vi "SE5082_Scaler.vi"(4 "Channel":u16(ring) items=["Channel 1", "Channel 2"], 8 "error in":errorcluster, 9 "Voffset":dbl, 10 "Vpp":dbl=1.0, 11 "VISA resource name in":refnum<visa-resource-name>="USB0::0x168C::0x5082::0000217419::INSTR") -> (0 "error out":errorcluster, 3 "VISA resource name out":refnum<visa-resource-name>="USB0::0x168C::0x5082::0000217419::INSTR")   [LabVIEW 2017]
uses:
  Software/Rydberg_Control/TypeDefinition/variables.ctl
panel:
  in  "HV_HI":string="200"
  in  "HV_LO":string="-100"
  in  "Readout status?":bool
  in  "Read-out commands":string[](array[string])=[":INST 1;:VOLT?", ":INST 1;:VOLT:OFFS?", ":INST 1;:OUTP?", ":INST 2;:VOLT?", ":INST 2;:VOLT:OFFS?", ":INST 2;:OUTP?"]
  out "Input waveform commands":string[](array[string])=[":INST 1;:OUTP OFF", ":INST 2;:OUTP OFF", ":INST 1;:VOLT  1.000000", ":INST 1;:VOLT:OFFS  -1.000000 "]
  out "Status output":string[](array[string])=["1.000e+00\n", "0.000e+00\n", "OFF\n", "5.000e-01\n", "0.000e+00\n", "OFF\n"]
  in  "Debug commands":string=":SOUR1:VOLT:OFFS 1\n:SOUR1:VOLT 6"
  in  "Variables":T1=[{"Value"=10.0, "Variable"="dummy", "Save with Image"=FALSE}, {"Value"=-0.0001, "Variable"="HI", "Save with Image"=FALSE}, {"Value"=-0.0002, "Variable"="LO", "Save with Image"=FALSE}, {"Value"=0.0, "Variable"="dummy1", "Save with Image"=FALSE}, {"Value"=0.0, "Variable"="dummy2", "Save with Image"=FALSE}, {"Value"=0.0, "Variable"="dummy3", "Save with Image"=FALSE}, {"Value"=0.0, "Variable"="tLEDuv", "Save with Image"=FALSE}, {"Value"=1000.0, "Variable"="tMOT0", "Save with Image"=FALSE}, {"Value"=20.0, "Variable"="tMOT1", "Save with Image"=FALSE}, {"Value"=40.0, "Variable"="tMOT2", "Save with Image"=FALSE}, {"Value"=50.0, "Variable"="tMOT3", "Save with Image"=FALSE}, {"Value"=13.0, "Variable"="tMOT3delayREP", "Save with Image"=FALSE}, {"Value"=0.05, "Variable"="tREP", "Save with Image"=FALSE}, {"Value"=0.75, "Variable"="dMOT0", "Save with Image"=FALSE}, {"Value"=1.75, "Variable"="dMOT1", "Save with Image"=FALSE}, {"Value"=1.75, "Variable"="dMOT2", "Save with Image"=FALSE}, {"Value"=0.0, "Variable"="dummy5", "Save with Image"=FALSE}, {"Value"=1.45, "Variable"="pMOT0", "Save with Image"=FALSE}, {"Value"=1.45, "Variable"="pMOT1", "Save with Image"=FALSE}, {"Value"=1.25, "Variable"="pMOT2", "Save with Image"=FALSE}, {"Value"=-1.0, "Variable"="dummy6", "Save with Image"=FALSE}, {"Value"=1.6, "Variable"="pRP0", "Save with Image"=FALSE}, {"Value"=1.6, "Variable"="pRP1", "Save with Image"=FALSE}, {"Value"=0.8, "Variable"="pRP2", "Save with Image"=FALSE}, {"Value"=0.0, "Variable"="MOTdummy0", "Save with Image"=FALSE}, {"Value"=-1.0, "Variable"="MOTdummy1", "Save with Image"=FALSE}, {"Value"=0.0, "Variable"="MOTdummy2", "Save with Image"=FALSE}, {"Value"=0.0, "Variable"="MOTdummy3", "Save with Image"=FALSE}, {"Value"=0.0, "Variable"="MOTdummy4", "Save with Image"=FALSE}, {"Value"=1.8, "Variable"="pCROSS0", "Save with Image"=FALSE}, {"Value"=1.29, "Variable"="pCROSS1", "Save with Image"=FALSE}, {"Value"=1.05, "Variable"="pCROSS2", "Save with Image"=FALSE}, {"Value"=0.75, "Variable"="pCROSS3", "Save with Image"=FALSE}, {"Value"=0.0, "Variable"="pCROSS4", "Save with Image"=FALSE}, {"Value"=5.0, "Variable"="pDIMPL0", "Save with Image"=FALSE}, {"Value"=4.4, "Variable"="pDIMPL1", "Save with Image"=FALSE}, {"Value"=3.65, "Variable"="pDIMPL2", "Save with Image"=FALSE}, {"Value"=3.55, "Variable"="pDIMPL3", "Save with Image"=FALSE}, {"Value"=3.45, "Variable"="pDIMPL4", "Save with Image"=FALSE}, {"Value"=1.8, "Variable"="pTightTrap", "Save with Image"=FALSE}, {"Value"=400.0, "Variable"="tHOLD", "Save with Image"=FALSE}, {"Value"=740.0, "Variable"="tEVAP1", "Save with Image"=FALSE}, {"Value"=2900.0, "Variable"="tEVAP2", "Save with Image"=FALSE}, {"Value"=590.0, "Variable"="tEVAP3", "Save with Image"=FALSE}, {"Value"=50.0, "Variable"="tEVAP4", "Save with Image"=FALSE}, {"Value"=50.0, "Variable"="tHOLDTight", "Save with Image"=FALSE}, {"Value"=0.0, "Variable"="ODTdummy1", "Save with Image"=FALSE}, {"Value"=0.0, "Variable"="ODTdummy2", "Save with Image"=FALSE}, {"Value"=0.0, "Variable"="ODTdummy3", "Save with Image"=FALSE}, {"Value"=0.0, "Variable"="ODTdummy4", "Save with Image"=FALSE}, {"Value"=0.0, "Variable"="ODTdummy5", "Save with Image"=FALSE}, {"Value"=3.59, "Variable"="dIMGx", "Save with Image"=FALSE}, {"Value"=3.59, "Variable"="dIMGx0", "Save with Image"=FALSE}, {"Value"=1.38, "Variable"="dIMGz", "Save with Image"=FALSE}, {"Value"=1.98, "Variable"="dEXCz", "Save with Image"=FALSE}, {"Value"=3.0, "Variable"="pABSx", "Save with Image"=FALSE}, {"Value"=1.35, "Variable"="pABSz", "Save with Image"=FALSE}, {"Value"=0.55, "Variable"="pEXCz", "Save with Image"=FALSE}, {"Value"=0.0, "Variable"="TOF", "Save with Image"=FALSE}, {"Value"=10.0, "Variable"="TOFatomFall", "Save with Image"=FALSE}, {"Value"=0.012, "Variable"="tEXP", "Save with Image"=FALSE}, {"Value"=0.2, "Variable"="tEXP2", "Save with Image"=FALSE}, {"Value"=0.082, "Variable"="tEXC", "Save with Image"=FALSE}, {"Value"=0.001, "Variable"="tWaitIoniz", "Save with Image"=FALSE}, {"Value"=0.065, "Variable"="tCAM", "Save with Image"=FALSE}, {"Value"=200.0, "Variable"="tCAMguppy", "Save with Image"=FALSE}, {"Value"=50.0, "Variable"="tCAMreadout", "Save with Image"=FALSE}, {"Value"=-0.002, "Variable"="tTrigDelay", "Save with Image"=FALSE}, {"Value"=0.0, "Variable"="tTrans", "Save with Image"=FALSE}, {"Value"=1.0, "Variable"="tEXCres", "Save with Image"=FALSE}, {"Value"=0.004, "Variable"="tPUMP", "Save with Image"=FALSE}, {"Value"=2.0, "Variable"="pBLUEswitch", "Save with Image"=FALSE}, {"Value"=2.0, "Variable"="pBLUEswitchEIT", "Save with Image"=FALSE}, {"Value"=3.5, "Variable"="dBLUE", "Save with Image"=FALSE}, {"Value"=3.5, "Variable"="dBLUE0", "Save with Image"=FALSE}, {"Value"=1.7, "Variable"="dBLUEdec", "Save with Image"=FALSE}, {"Value"=2.5, "Variable"="dBLUEdec0", "Save with Image"=FALSE}, {"Value"=3.2, "Variable"="dIMPnew", "Save with Image"=FALSE}, {"Value"=1.0, "Variable"="blueON1", "Save with Image"=FALSE}, {"Value"=0.0, "Variable"="blueON2", "Save with Image"=FALSE}, {"Value"=1.0, "Variable"="blueEXCON1", "Save with Image"=FALSE}, {"Value"=0.0, "Variable"="blueEXCON2", "Save with Image"=FALSE}, {"Value"=35.637858, "Variable"="dRydMW", "Save with Image"=FALSE}, {"Value"=16.0, "Variable"="pRydMW", "Save with Image"=FALSE}, {"Value"=50.0, "Variable"="MWduration", "Save with Image"=FALSE}, {"Value"=4.33, "Variable"="bmw0", "Save with Image"=FALSE}, {"Value"=0.02, "Variable"="bmw1", "Save with Image"=FALSE}, {"Value"=0.0, "Variable"="MWdummy1", "Save with Image"=FALSE}, {"Value"=0.0, "Variable"="MWdummy2", "Save with Image"=FALSE}, {"Value"=0.0, "Variable"="MWdummy3", "Save with Image"=FALSE}, {"Value"=4.3, "Variable"="foffset", "Save with Image"=FALSE}, {"Value"=8.64, "Variable"="fdx", "Save with Image"=FALSE}, {"Value"=-5.78, "Variable"="fdy", "Save with Image"=FALSE}, {"Value"=4.0, "Variable"="fdz", "Save with Image"=FALSE}, {"Value"=300.0, "Variable"="CH203", "Save with Image"=FALSE}, {"Value"=160.0, "Variable"="CH215", "Save with Image"=FALSE}, {"Value"=4.0, "Variable"="CH302", "Save with Image"=FALSE}, {"Value"=280.0, "Variable"="CH315", "Save with Image"=FALSE}, {"Value"=0.0, "Variable"="CH202", "Save with Image"=FALSE}, {"Value"=0.0, "Variable"="CH308", "Save with Image"=FALSE}, {"Value"=0.0, "Variable"="EFIELDdummy2", "Save with Image"=FALSE}, {"Value"=0.0, "Variable"="EFIELDdummy3", "Save with Image"=FALSE}, {"Value"=0.0, "Variable"="EFIELDdummy4", "Save with Image"=FALSE}, {"Value"=0.0, "Variable"="EFIELDdummy5", "Save with Image"=FALSE}, {"Value"=0.0, "Variable"="EFIELDdummy6", "Save with Image"=FALSE}, {"Value"=0.0, "Variable"="EFIELDdummy7", "Save with Image"=FALSE}, {"Value"=1.25, "Variable"="bMOT0", "Save with Image"=FALSE}, {"Value"=2.5, "Variable"="bMOT1", "Save with Image"=FALSE}, {"Value"=2.5, "Variable"="bMOT2", "Save with Image"=FALSE}, {"Value"=1.25, "Variable"="bMOT3", "Save with Image"=FALSE}, {"Value"=0.0, "Variable"="bCOMPx", "Save with Image"=FALSE}, {"Value"=1.35, "Variable"="bCOMPy", "Save with Image"=FALSE}, {"Value"=0.27, "Variable"="bCOMPz", "Save with Image"=FALSE}, {"Value"=0.7, "Variable"="bCOMPx1", "Save with Image"=FALSE}, {"Value"=1.1, "Variable"="bCOMPy1", "Save with Image"=FALSE}, {"Value"=0.5, "Variable"="bCOMPz1", "Save with Image"=FALSE}, {"Value"=4.35, "Variable"="bxfinal", "Save with Image"=FALSE}, {"Value"=0.0, "Variable"="byfinal", "Save with Image"=FALSE}, {"Value"=0.0, "Variable"="bzfinal", "Save with Image"=FALSE}, {"Value"=0.0, "Variable"="BFIELDdummy1", "Save with Image"=FALSE}, {"Value"=0.0, "Variable"="BFIELDdummy2", "Save with Image"=FALSE}, {"Value"=0.0, "Variable"="BFIELDdummy3", "Save with Image"=FALSE}, {"Value"=10.0, "Variable"="tCOILsettle", "Save with Image"=FALSE}, {"Value"=0.0, "Variable"="tRemove", "Save with Image"=FALSE}, {"Value"=3.6, "Variable"="pRemove", "Save with Image"=FALSE}, {"Value"=3.1, "Variable"="dF2CLEAN1x", "Save with Image"=FALSE}, {"Value"=20.0, "Variable"="tF2CLEAN1x", "Save with Image"=FALSE}, {"Value"=4.0, "Variable"="tF2CLEAN2x", "Save with Image"=FALSE}, {"Value"=0.0, "Variable"="tDelayDown", "Save with Image"=FALSE}, {"Value"=156.0, "Variable"="oDDSbluePro", "Save with Image"=FALSE}, {"Value"=-10.25, "Variable"="dDDSbluePro", "Save with Image"=FALSE}, {"Value"=50.0, "Variable"="tRampDDSbluePro", "Save with Image"=FALSE}, {"Value"=416.6261, "Variable"="oDDSred", "Save with Image"=FALSE}, {"Value"=-50.25, "Variable"="dDDSred", "Save with Image"=FALSE}, {"Value"=90.0, "Variable"="tRampDDSred", "Save with Image"=FALSE}, {"Value"=154.0, "Variable"="oDDSblueOld", "Save with Image"=FALSE}, {"Value"=10.0, "Variable"="dDDSblueOld", "Save with Image"=FALSE}, {"Value"=100.0, "Variable"="tRampDDSblueOld", "Save with Image"=FALSE}, {"Value"=1.0, "Variable"="mwON", "Save with Image"=FALSE}, {"Value"=9.4e-05, "Variable"="tRabi", "Save with Image"=FALSE}, {"Value"=9.4e-05, "Variable"="tRabi2", "Save with Image"=FALSE}, {"Value"=5e-05, "Variable"="tRamsey", "Save with Image"=FALSE}, {"Value"=0.0, "Variable"="tRamsey2", "Save with Image"=FALSE}, {"Value"=0.0, "Variable"="tDDSa", "Save with Image"=FALSE}, {"Value"=0.0, "Variable"="tDDSb", "Save with Image"=FALSE}, {"Value"=399.942, "Variable"="dDDSa", "Save with Image"=FALSE}, {"Value"=399.942, "Variable"="dDDSa2", "Save with Image"=FALSE}, {"Value"=0.2, "Variable"="pDDSa", "Save with Image"=FALSE}, {"Value"=1e-07, "Variable"="pDDSa2", "Save with Image"=FALSE}, {"Value"=0.0, "Variable"="phiDDSa", "Save with Image"=FALSE}, {"Value"=0.875, "Variable"="phiDDSa2", "Save with Image"=FALSE}, {"Value"=399.942, "Variable"="dDDSb", "Save with Image"=FALSE}, {"Value"=400.009, "Variable"="dDDSb2", "Save with Image"=FALSE}, {"Value"=0.25, "Variable"="pDDSb", "Save with Image"=FALSE}, {"Value"=1e-07, "Variable"="pDDSb2", "Save with Image"=FALSE}, {"Value"=0.25, "Variable"="phiDDSb", "Save with Image"=FALSE}, {"Value"=0.55, "Variable"="phiDDSb2", "Save with Image"=FALSE}, {"Value"=300.0, "Variable"="tDipole", "Save with Image"=FALSE}, {"Value"=0.7, "Variable"="bCOMPx2", "Save with Image"=FALSE}, {"Value"=0.8, "Variable"="bCOMPy2", "Save with Image"=FALSE}, {"Value"=0.6, "Variable"="bCOMPz2", "Save with Image"=FALSE}, {"Value"=20.0, "Variable"="dMOTRamp1", "Save with Image"=FALSE}, {"Value"=18.0, "Variable"="DMOTload", "Save with Image"=FALSE}, {"Value"=50.0, "Variable"="dMOTRamp2", "Save with Image"=FALSE}, {"Value"=272.0, "Variable"="DMOTimag", "Save with Image"=FALSE}, {"Value"=1000.0, "Variable"="oDDShyperfine", "Save with Image"=FALSE}, {"Value"=0.1, "Variable"="dDDShyperfine", "Save with Image"=FALSE}, {"Value"=0.0, "Variable"="tof", "Save with Image"=FALSE}, {"Value"=262.5, "Variable"="dOPump", "Save with Image"=FALSE}, {"Value"=4500.0, "Variable"="tRampOPump", "Save with Image"=FALSE}, {"Value"=10.0, "Variable"="tOPump", "Save with Image"=FALSE}, {"Value"=1.5, "Variable"="bCOMPx3", "Save with Image"=FALSE}, {"Value"=0.8, "Variable"="bCOMPy3", "Save with Image"=FALSE}, {"Value"=0.0, "Variable"="bCOMPz3", "Save with Image"=FALSE}, {"Value"=0.0, "Variable"="bCOMPx4", "Save with Image"=FALSE}, {"Value"=0.0, "Variable"="bCOMPy4", "Save with Image"=FALSE}, {"Value"=0.0, "Variable"="bCOMPz4", "Save with Image"=FALSE}, {"Value"=0.0, "Variable"="scan2photRes", "Save with Image"=FALSE}, {"Value"=0.0, "Variable"="tEXCsmallProbe", "Save with Image"=FALSE}, {"Value"=0.082, "Variable"="tEXCBlue", "Save with Image"=FALSE}, {"Value"=0.0015, "Variable"="tDownPump", "Save with Image"=FALSE}, {"Value"=98.75, "Variable"="RF1freq1", "Save with Image"=FALSE}, {"Value"=0.1, "Variable"="RF1freq2", "Save with Image"=FALSE}, {"Value"=98.75, "Variable"="dummya", "Save with Image"=FALSE}, {"Value"=0.1, "Variable"="dummyb", "Save with Image"=FALSE}] {"Value" format="%#.9g"}
  # "Vpp define peak-to-peak value, Voffset define offset value"
  # "100e-3 to +1.2"
  # "DC: -0. 5 to +0.5"
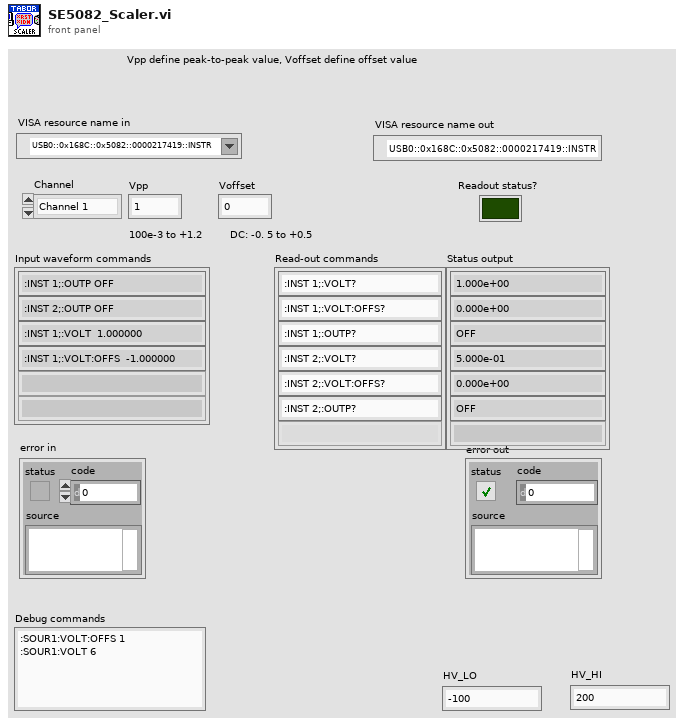
[diagram p1: front panel]
types:
  T1 = typedef "variables.ctl" = cluster{"Value":dbl, "Variable":string, "Save with Image":bool}[]
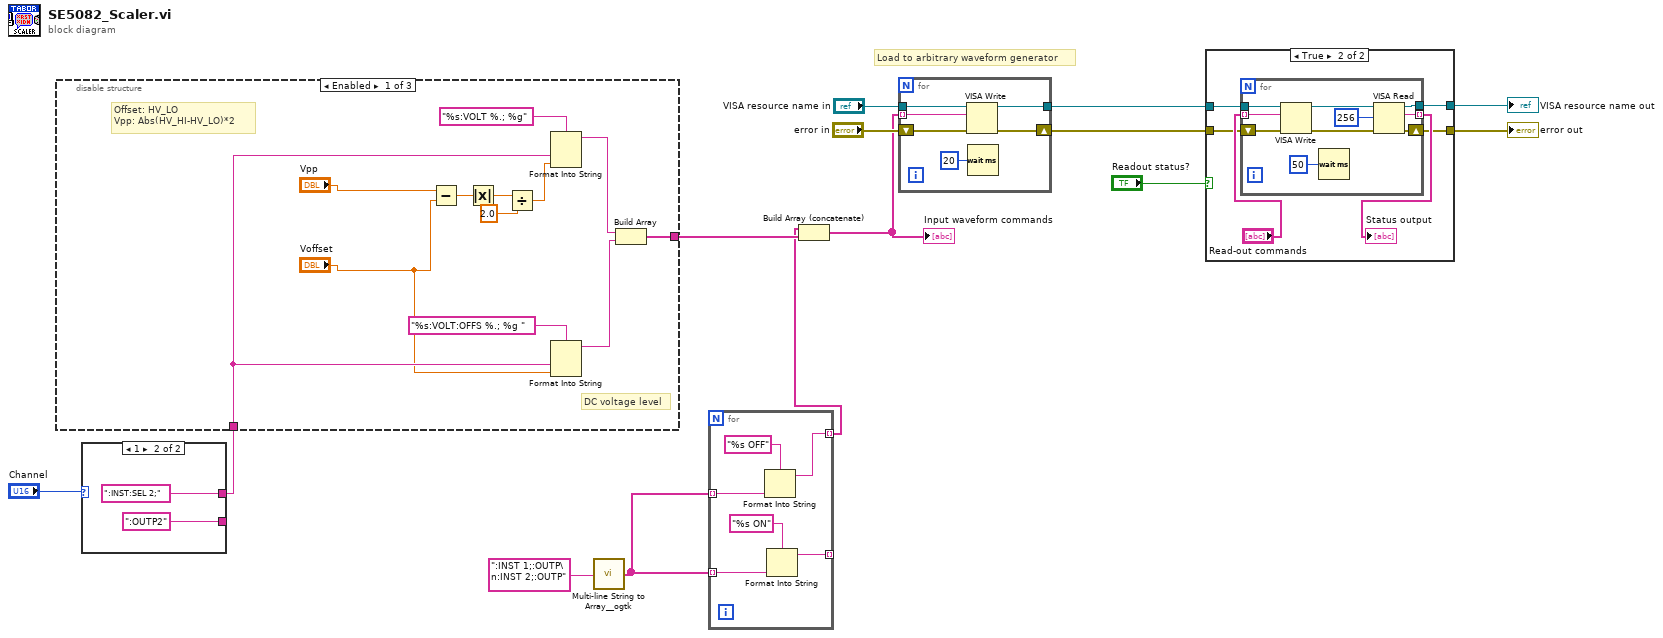
[diagram p0: block diagram]
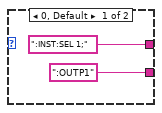
[diagram p2: hidden frame]
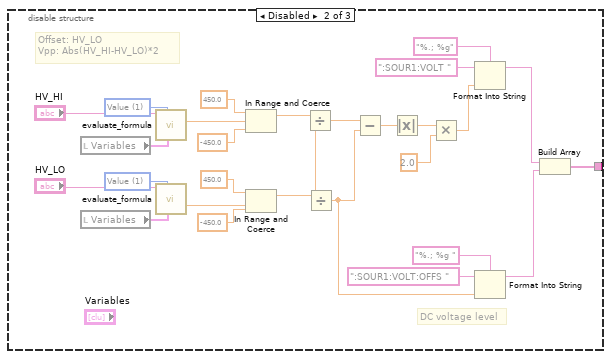
[diagram p4: hidden frame]
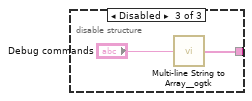
[diagram p5: hidden frame]
diagram:
  # "Load to arbitrary waveform generator"
  n1 = case shown="1" "Channel" {
    tunnel: [":INST:SEL 1;" ("initial string") ":INST:SEL 2;" ("initial string")] -> w4
    tunnel: [":OUTP1" ("initial string") ":OUTP2" ("initial string")] -> _
    frame 0, Default {
    }
    frame 1 {
    }
  }
  n2 = disable-structure shown="Enabled" {
    disable-tunnel: [w28 w41 w59] -> w11
    disable-tunnel: w4 -> [w22 _ _]
    frame Enabled {
      # "Offset: HV_LO\nVpp: Abs(HV_HI-HV_LO)*2"
      # "DC voltage level"
      n3 = Subtract(x="Vpp", y="Voffset") -> (x-y=w25:dbl)
      n4 = Absolute Value(x=w25) -> (abs(x)=w24:dbl)
      n5 = Divide(x=w24, y=2.0) -> (x/y=w23:dbl)
      n6 = Format Into String(format string="%s:VOLT %.; %g", w22, w23) -> (resulting string=w26:string)  [unwired: 2 in, 1 out]
      n7 = Format Into String(format string="%s:VOLT:OFFS %.; %g ", w22, "Voffset") -> (resulting string=w29:string)  [unwired: 2 in, 1 out]
      n8 = Build Array(w26, w29) -> (w28:string[])
    }
    frame Disabled {
      w55 = u16 1 items=["Time in counts", "Value"] ("Time or Value")
      w58 = u16 1 items=["Time in counts", "Value"] ("Time or Value")
      # "Offset: HV_LO\nVpp: Abs(HV_HI-HV_LO)*2"
      # "DC voltage level"
      n9 = local read "Variables"() -> (w57:T1)
      n10 = local read "Variables"() -> (w56:T1)
      n11 = call "evaluate_formula.vi"("Variable array"=w57, "Time or Value"=w58, "Formula"="HV_HI") -> ("Output"=w48:dbl)  [unwired: 7 in, 1 out]
      n12 = call "evaluate_formula.vi"("Variable array"=w56, "Time or Value"=w55, "Formula"="HV_LO") -> ("Output"=w47:dbl)  [unwired: 7 in, 1 out]
      n13 = In Range and Coerce(upper limit=450.0, x=w48, lower limit=-450.0) -> (coerced(x)=w46:dbl)  [unwired: 1 out]
      n14 = In Range and Coerce(upper limit=450.0, x=w47, lower limit=-450.0) -> (coerced(x)=w45:dbl)  [unwired: 1 out]
      n15 = Divide(x=w46) -> (y=w31:dbl, x/y=w36:dbl)
      n16 = Divide(x=w45, y=w31) -> (x/y=w35:dbl)
      n17 = Subtract(x=w36, y=w35) -> (x-y=w37:dbl)
      n18 = Absolute Value(x=w37) -> (abs(x)=w34:dbl)
      n19 = Multiply(x=w34, y=2.0) -> (x*y=w32:dbl)
      n20 = Format Into String(format string="%.; %g", initial string=":SOUR1:VOLT ", w32) -> (resulting string=w38:string)  [unwired: 1 in, 1 out]
      n21 = Format Into String(format string="%.; %g ", initial string=":SOUR1:VOLT:OFFS ", w35) -> (resulting string=w42:string)  [unwired: 1 in, 1 out]
      n22 = Build Array(w38, w42) -> (w41:string[])
    }
    frame Disabled {
      n23 = call <userlib>:"Multi-line String to Array__ogtk.vi"("string"="Debug commands") -> ("lines"=w59:string[])
    }
  }
  n24 = call <userlib>:"Multi-line String to Array__ogtk.vi"("string"=":INST 1;:OUTP\n:INST 2;:OUTP" ("initial string")) -> ("lines"=w1:string[])
  n25 = for {
    tunnel: w1 -> [w64] mode=indexing
    tunnel: [w65] -> w3 mode=indexing
    tunnel: w1 -> [w62] mode=indexing
    tunnel: [w61] -> _ mode=indexing
    n26 = Format Into String(format string="%s OFF", w64) -> (resulting string=w65:string)  [unwired: 2 in, 1 out]
    n27 = Format Into String(format string="%s ON", w62) -> (resulting string=w61:string)  [unwired: 2 in, 1 out]
  }
  n28 = Build Array (concatenate)(w3, w11) -> (w12:string[])
  "Input waveform commands" <- w12
  n29 = for {
    tunnel: "VISA resource name in" -> [w72]
    tunnel: w12 -> [w71] mode=indexing
    shift-right: [w69] -> w9
    shift-left: "error in" -> [w70]
    tunnel: [w68] -> w10
    n30 = VISA Write(VISA resource name=w72, write buffer=w71, error in (no error)=w70) -> (VISA resource name out=w68:refnum<visa-resource-name>, error out=w69:errorcluster)  [unwired: 1 out]
    n31 = Wait (ms)(milliseconds to wait=u32 20) -> ()  [unwired: 1 out]
  }
  n32 = case shown="True" "Readout status?" {
    tunnel: w10 -> [w74 w78]
    tunnel: w9 -> [w73 w77]
    tunnel: [w73 w76] -> w8
    tunnel: [w74 w75] -> w7
    frame False {
    }
    frame True {
      n33 = for {
        tunnel: [w87] -> w80 mode=indexing
        shift-right: [w86] -> w76
        shift-left: w77 -> [w83]
        tunnel: w78 -> [w85]
        tunnel: "Read-out commands" -> [w84] mode=indexing
        tunnel: [w81] -> w75
        n34 = VISA Write(VISA resource name=w85, write buffer=w84, error in (no error)=w83) -> (VISA resource name out=w89:refnum<visa-resource-name>, error out=w88:errorcluster)  [unwired: 1 out]
        n35 = Wait (ms)(milliseconds to wait=u32 50) -> ()  [unwired: 1 out]
        n36 = VISA Read(VISA resource name=w89, byte count=u32 256, error in (no error)=w88) -> (VISA resource name out=w81:refnum<visa-resource-name>, read buffer=w87:string, error out=w86:errorcluster)  [unwired: 1 out]
      }
      "Status output" <- w80
    }
  }
  "error out" <- w8
  "VISA resource name out" <- w7
